vi "Bake.vi"(8 "error in (no error)":errorcluster, 11 "Appliance in":refnum<class "Appliance.lvclass">) -> (0 "error out":errorcluster, 3 "Appliance out":refnum<class "Appliance.lvclass">)   [LabVIEW 2011, in "Appliance.lvclass"]
uses:
  Appliance.lvclass
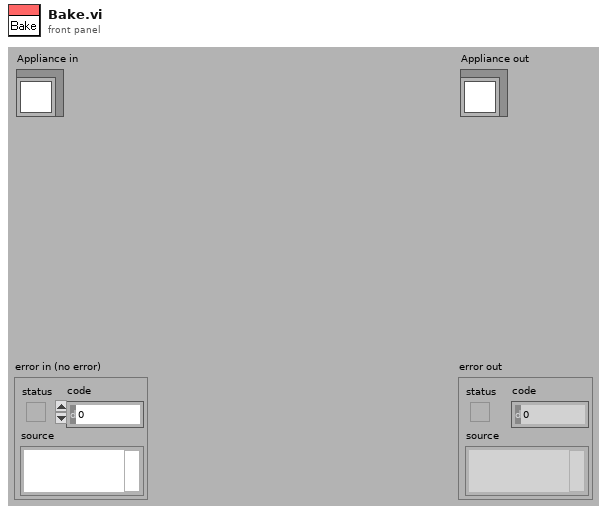
[diagram p1: front panel]
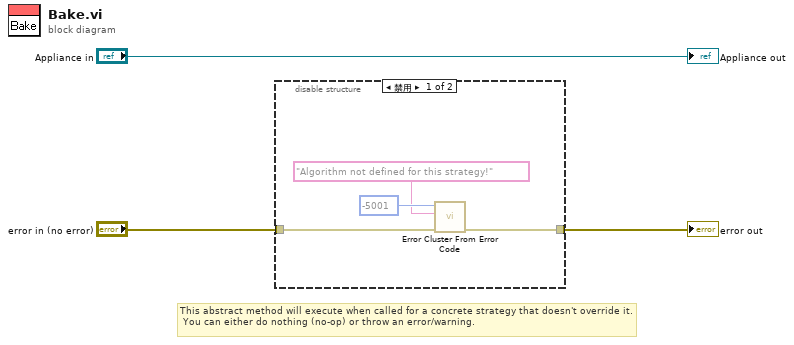
[diagram p0: block diagram]
diagram:
  # "This abstract method will execute when called for a concrete strategy that doesn't override it.\n You can either do nothing (no-op) or throw an error/warning."
  n1 = disable-structure shown="禁用" {
    disable-tunnel: "error in (no error)" -> [w7 w8]
    disable-tunnel: [w6 w8] -> w1
    frame Disabled {
      n2 = call <vilib>:"Error Cluster From Error Code.vi"("error in (no error)"=w7, "error message (\"\")"="Algorithm not defined for this strategy!" ("error message (\"\")"), "error code (0)"=-5001) -> ("error out"=w6:errorcluster)  [unwired: 6 in]
    }
    frame Enabled {
    }
  }
  "error out" <- w1
  "Appliance out" <- "Appliance in"
